vi "Create API Case in Message Handler.vi"(8 "error in (no error)":errorcluster, 11 "Setter Generator In":refnum<class "API VI Generator.lvclass">) -> (0 "error out":errorcluster, 3 "Setter Generator Out":refnum<class "API VI Generator.lvclass">)   [LabVIEW 2020, in "Method Generation.lvlib" / "API VI Generator.lvclass"]
uses:
  API VI Generator.lvclass
  <vilib>/Utility/traverseref.llb/TRef TravTarget.ctl
  API VI Generator.lvclass/API VI Generator.ctl
  <vilib>/Utility/miscctls.llb/LVPointTypeDef.ctl
  <vilib>/Utility/traverseref.llb/VI Scripting - Traverse.lvlib
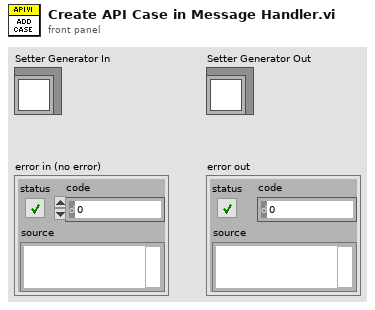
[diagram p1: front panel]
types:
  T1 = typedef "TRef TravTarget.ctl" = enum16{"FP", "BD", "Other"}
  T2 = typedef "LVPointTypeDef.ctl" = cluster{"Horizontal":i16, "Vertical":i16}
  T3 = typedef "LVBoundsTypeDef.ctl" = cluster{"Width":u32, "Height":u32}
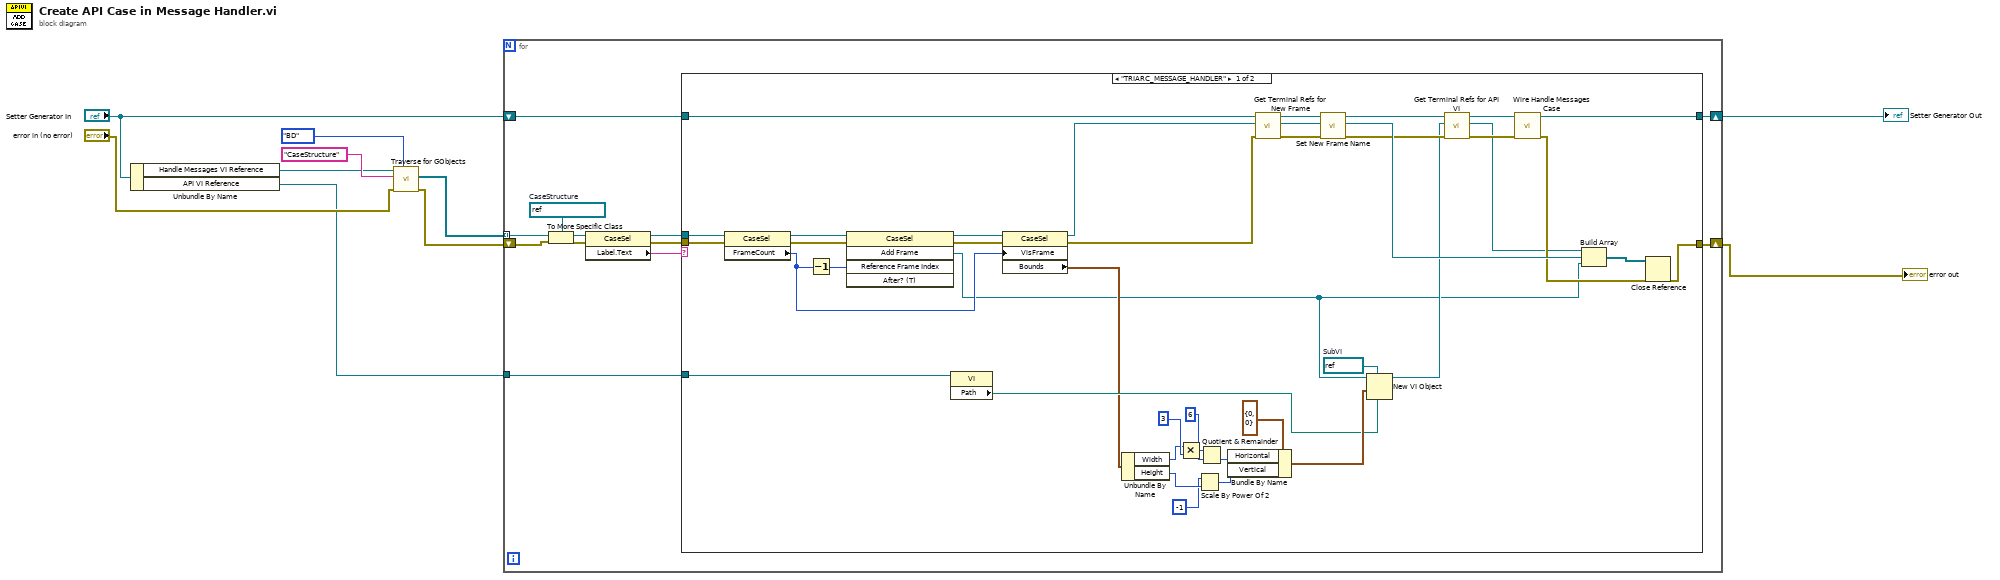
[diagram p0: block diagram]
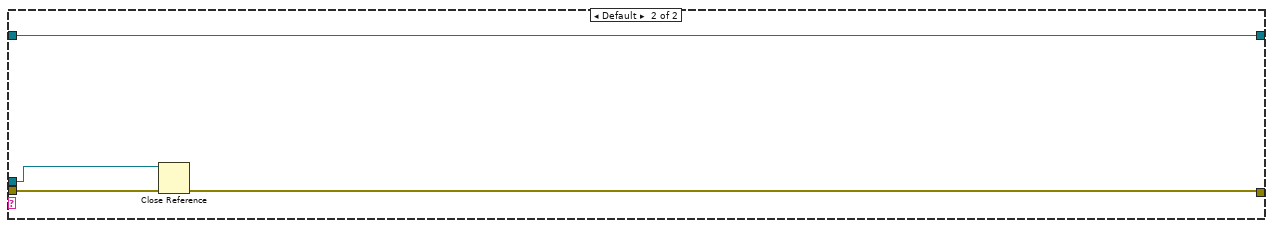
[diagram p2: hidden frame]
diagram:
  n1 = Unbundle By Name("Setter Generator In") -> ("Handle Messages VI Reference"=w2:refnum<vi>, "API VI Reference"=w1:refnum<vi>)
  n2 = call <vilib>:"Traverse for GObjects.vi"("Traverse Target"=TRef_TravTarget."BD", "error in (no error)"="error in (no error)", "Class Name"="CaseStructure", "VI Refnum"=w2) -> ("error out"=w3:errorcluster, "References"=w5:refnum<vi>[])  [unwired: 4 in, 2 out]
  n3 = for {
    tunnel: w5 -> [w20] mode=indexing
    shift-right: [w14] -> w4
    shift-left: w3 -> [w17]
    shift-right: [w12] -> w7
    shift-left: "Setter Generator In" -> [w13]
    tunnel: w1 -> [w11]
    w16 = refnum<vi> refnum  # CaseStructure
    n4 = To More Specific Class(target class=w16, reference=w20, error in=w17) -> (specific class reference=w19:refnum<vi>, error out=w18:errorcluster)
    n5 = property class="CaseSel"(reference=w19, error in=w18) -> (reference out=w21:refnum<vi>, error out=w15:errorcluster, "Label.Text"=w22:string)
    n6 = case shown="\"TRIARC_MESSAGE_HANDLER\"" w22 {
      tunnel: w21 -> [w50 w66]
      tunnel: w15 -> [w49 w65]
      tunnel: [w59 w64] -> w14
      tunnel: w13 -> [w62 w63]
      tunnel: [w27 w63] -> w12
      tunnel: w11 -> [w31 _]
      frame "TRIARC_MESSAGE_HANDLER" {
        w29 = refnum<vi> refnum  # SubVI
        n7 = property class="CaseSel"(reference=w50, error in=w49) -> (reference out=w51:refnum<vi>, error out=w48:errorcluster, "FrameCount"=w46:i32)
        n8 = Decrement(x=w46) -> (x-1=w47:i32)
        n9 = invoke class="CaseSel" method="Add Frame"(reference=w51, error in=w48, "Reference Frame Index"=w47) -> (reference out=w53:refnum<vi>, error out=w52:errorcluster, "Add Frame"=w23:refnum<vi>)  [unwired: 2 in, 2 out]
        n10 = property class="VI"(reference=w31) -> ("Path"=w35:path)  [unwired: 1 in, 2 out]
        n11 = property class="CaseSel"(reference=w53, error in=w52, "VisFrame"=w46) -> (reference out=w34:refnum<vi>, error out=w33:errorcluster, "Bounds"=w32:T3)
        n12 = Unbundle By Name(w32) -> ("Width"=w37:u32, "Height"=w45:u32)
        n13 = Multiply(x=w37, y=u32 3) -> (x*y=w39:u32)
        n14 = Scale By Power Of 2(n=i16 -1, x=w45) -> (x*2^n=w42:u32)
        n15 = Quotient & Remainder(x=w39, y=u32 6) -> (floor(x/y)=w43:u32)  [unwired: 1 out]
        n16 = Bundle By Name(cluster=T2 {"Horizontal"=0, "Vertical"=0} ("location"), "Horizontal"=w43, "Vertical"=w42) -> (w36:T2)
        n17 = call "Get Terminal Refs for New Frame.vi"("error in (no error)"=w33, "Case Structure Ref"=w34, "Setter Generator In"=w62) -> ("error out"=w56:errorcluster, "reference out"=w58:refnum<vi>, "Setter Generator Out"=w61:refnum<class "API VI Generator.lvclass">)  [unwired: 6 in]
        n18 = call "Set New Frame Name.vi"("error in (no error)"=w56, "reference in"=w58, "Setter Generator In"=w61) -> ("error out"=w55:errorcluster, "reference out"=w57:refnum<vi>, "Setter Generator Out"=w54:refnum<class "API VI Generator.lvclass">)  [unwired: 6 in]
        n19 = New VI Object(vi object class=w29, owner refnum=w23, position/next to=w36, 6:w35) -> (object refnum=w30:refnum<vi>)  [unwired: 4 in, 1 out]
        n20 = call "Get Terminal Refs for API VI.vi"("error in (no error)"=w55, "SubVI ref"=w30, "Setter Generator In"=w54) -> ("error out"=w26:errorcluster, "SubVI ref out"=w24:refnum<vi>, "Setter Generator Out"=w28:refnum<class "API VI Generator.lvclass">)  [unwired: 6 in]
        n21 = call "Wire Handle Messages Case.vi"("error in (no error)"=w26, "Setter Generator In"=w28) -> ("error out"=w25:errorcluster, "Setter Generator Out"=w27:refnum<class "API VI Generator.lvclass">)  [unwired: 8 in]
        n22 = Build Array(w24, w57, w23) -> (w60:refnum<vi>[])
        n23 = Close Reference(reference=w60, error in (no error)=w25) -> (error out=w59:errorcluster)
      }
      frame Default {
        n24 = Close Reference(reference=w66, error in (no error)=w65) -> (error out=w64:errorcluster)
      }
    }
  }
  "Setter Generator Out" <- w7
  "error out" <- w4
